vi "ClimatronicsUDP_get_rdg.vi"(4 "Channel Name":string, 7 "Address":T1={"Main"=61557, "Ch."=0, "Sub"=982, "Port Name"=""}) -> (0 "Output":dbl format="%.2f", 3 "Status note":string)   [LabVIEW 2011]
uses:
  ADAM Client/Sub VIs/ADAM Controls/Address.ctl
  ADAM Client/Sub VIs/ADAM Controls/Remember_value_mode.ctl
panel:
  out "error out 2":errorcluster
  out "error out":errorcluster
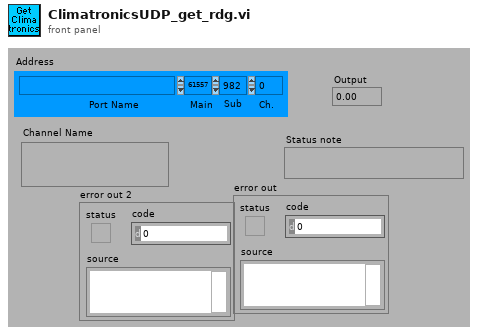
[diagram p1: front panel]
types:
  T1 = typedef "Address.ctl" = cluster{"Main":i32, "Ch.":i32, "Sub":i32, "Port Name":string}
  T2 = typedef "Remember_value_mode.ctl" = enum16{"Read only", "Read and Write"}
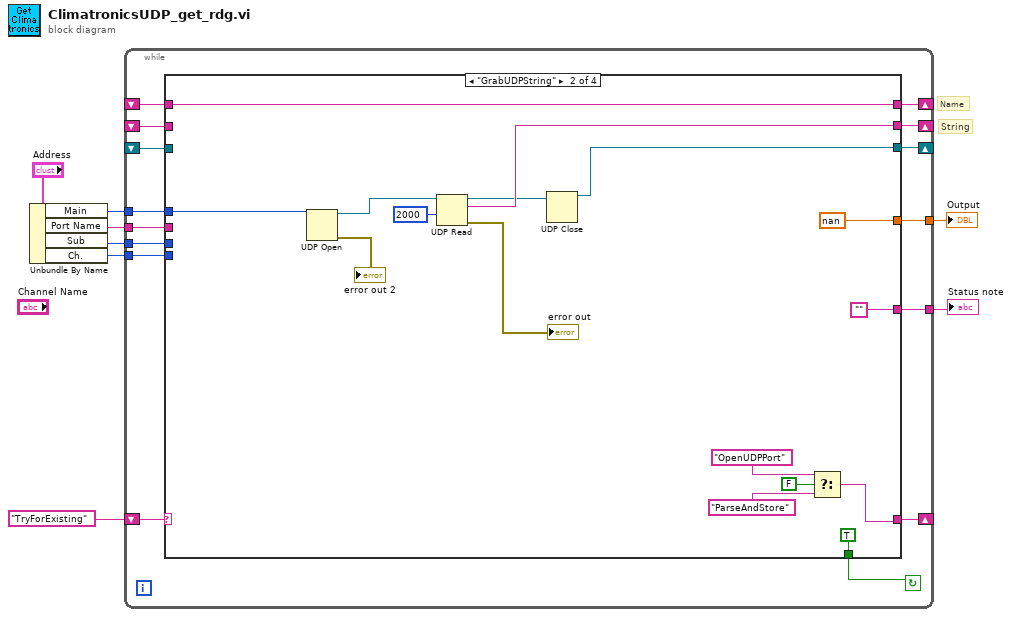
[diagram p0: block diagram]
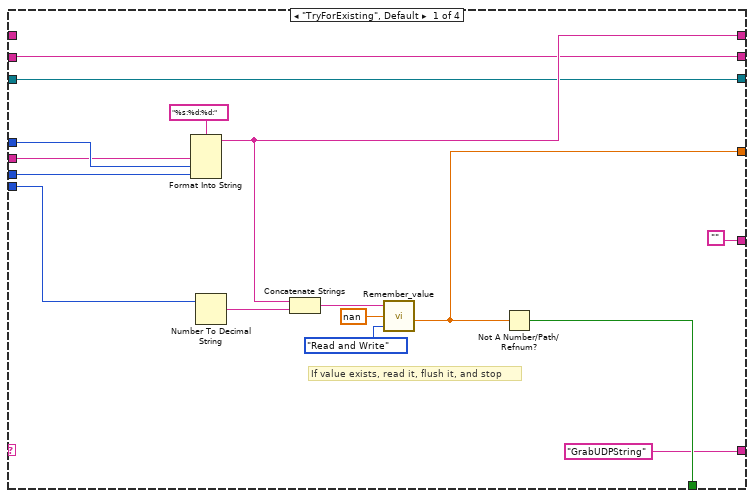
[diagram p2: hidden frame]
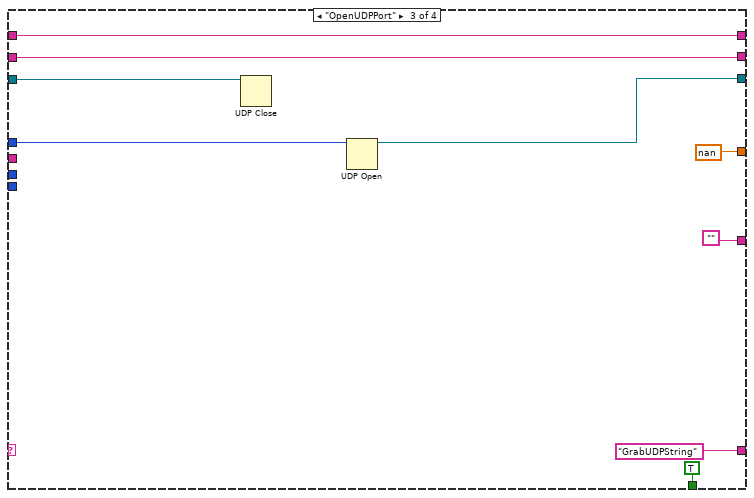
[diagram p3: hidden frame]
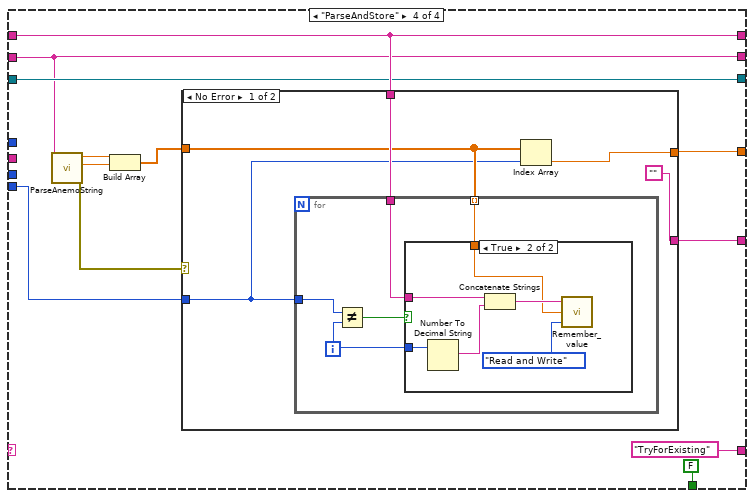
[diagram p4: hidden frame]
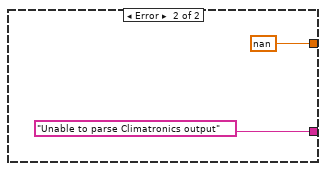
[diagram p6: hidden frame]
diagram:
  # "String"
  # "Name"
  n1 = Unbundle By Name("Address") -> ("Main"=w2:i32, "Port Name"=w7:string, "Sub"=w6:i32, "Ch."=w3:i32)
  n2 = while {
    shift-left: _ -> [w11]
    shift-right: [w12] -> _
    shift-left: _ -> [w14]
    shift-right: [w15] -> _
    tunnel: [w17] -> w4
    tunnel: [w18] -> w5
    shift-left: _ -> [w13]
    shift-right: [w19] -> _
    shift-left: "TryForExisting" -> [w10]
    shift-right: [w9] -> _
    tunnel: w3 -> [w20]
    tunnel: w2 -> [w21]
    tunnel: w6 -> [w22]
    tunnel: w7 -> [w23]
    stop <- w16 continue-if-true
    n3 = case shown="\"GrabUDPString\"" w10 {
      tunnel: w23 -> [w26 _ _ _]
      tunnel: w22 -> [w38 _ _ _]
      tunnel: w21 -> [w39 w46 w62 _]
      tunnel: w20 -> [w36 _ _ w74]
      tunnel: ["GrabUDPString" w49 "GrabUDPString" "TryForExisting"] -> w9
      tunnel: [w35 w54 w60 w73] -> w19
      tunnel: [w28 nan nan w75] -> w18
      tunnel: ["" "" "" w65] -> w17
      tunnel: [w27 TRUE TRUE FALSE] -> w16
      tunnel: [w30 w53 w59 w71] -> w15
      tunnel: w14 -> [w30 _ w59 w71]
      tunnel: w13 -> [_ w54 w60 w73]
      tunnel: [w25 w40 w64 w72] -> w12
      tunnel: w11 -> [w25 _ w63 w72]
      frame "TryForExisting", Default {
        # "If value exists, read it, flush it, and stop"
        n4 = Format Into String(format string="%s:%d:%d:" ("Format String"), w26, w39, w38) -> (resulting string=w35:string)  [unwired: 2 in, 1 out]
        n5 = Number To Decimal String(number=w36) -> (decimal integer string=w34:string)  [unwired: 1 out]
        n6 = Concatenate Strings(w35, w34) -> (w33:string)
        n7 = call "Remember_value.vi"("Mode"=Remember_value_mode."Read and Write", "Input Value"=nan, "Ch name"=w33) -> ("Output Value"=w28:dbl)
        n8 = Not A Number/Path/Refnum?(number/path/refnum=w28) -> (NaN/Path/Refnum?=w27:bool)
      }
      frame "GrabUDPString" {
        n9 = UDP Open(11:w46) -> (port=w45:refnum<k16>, 0:→"error out 2":errorcluster)  [unwired: 4 in, 1 out]
        n10 = UDP Read(connection ID=w45, timeout ms (25000)=2000) -> (data out=w53:string, error out=→"error out":errorcluster, 3:w41:refnum<k16>)  [unwired: 2 in, 2 out]
        n11 = UDP Close(connection ID=w41) -> (connection ID out=w40:refnum<k16>)  [unwired: 1 in, 1 out]
        n12 = Select(t="OpenUDPPort", s=FALSE, f="ParseAndStore") -> (s? t:f=w49:string)
      }
      frame "OpenUDPPort" {
        n13 = UDP Close(connection ID=w63) -> ()  [unwired: 1 in, 2 out]
        n14 = UDP Open(11:w62) -> (port=w64:refnum<k16>)  [unwired: 4 in, 2 out]
      }
      frame "ParseAndStore" {
        n15 = call "ParseAnemoString.vi"("String"=w71) -> ("error out"=w66:errorcluster, "direction"=w68:dbl, "speed"=w69:dbl)  [unwired: 8 in]
        n16 = Build Array(w69, w68) -> (w67:dbl[])
        n17 = case shown="No Error" w66 {
          tunnel: w67 -> [w79 _]
          tunnel: [w81 nan] -> w75
          tunnel: w74 -> [w78 _]
          tunnel: w73 -> [w80 _]
          tunnel: ["" "Unable to parse Climatronics output"] -> w65
          frame No Error {
            n18 = for {
              tunnel: w80 -> [w86]
              tunnel: w79 -> [w85] mode=indexing
              tunnel: w78 -> [w83]
              i -> [w84]
              n19 = Not Equal?(x=w83, y=w84) -> (x != y?=w82:bool)
              n20 = case shown="True" w82 {
                tunnel: w84 -> [_ w92]
                tunnel: w86 -> [_ w90]
                tunnel: w85 -> [_ w87]
                frame False {
                }
                frame True {
                  n21 = Number To Decimal String(number=w92) -> (decimal integer string=w91:string)  [unwired: 1 out]
                  n22 = Concatenate Strings(w90, w91) -> (w88:string)
                  n23 = call "Remember_value.vi"("Mode"=Remember_value_mode."Read and Write", "Input Value"=w87, "Ch name"=w88) -> ()  [unwired: 1 out]
                }
              }
            }
            n24 = Index Array(array=w79, index=w78) -> (element=w81:dbl)
          }
          frame Error {
          }
        }
      }
    }
  }
  "Output" <- w5
  "Status note" <- w4
